vi "Create Measure VI for Client.vi"(7 "client service_class":string, 8 "error in":errorcluster, 9 "results data":T1[](array[typedef]), 10 "configuration data":T4[](array[typedef]), 11 "measure vi refnum":refnum<vi>) -> (0 "error out":errorcluster)   [LabVIEW 2021, in "MeasurementClient Editor.lvlib"]
uses:
  MeasurementClient Editor.lvlib
  <vilib>/gRPC/Generated APIs/ni/measurementlink/measurement/v2/Measurement Service Client/RPC Messages/ni_measurementlink_measurement_v2_ConfigurationParameter.ctl
  <vilib>/gRPC/Generated APIs/ni/measurementlink/measurement/v2/Measurement Service Client/RPC Messages/google_protobuf_Field_Kind.ctl
  <vilib>/gRPC/Generated APIs/ni/measurementlink/measurement/v2/Measurement Service Client/RPC Messages/ni_measurementlink_measurement_v2_ConfigurationParameter_AnnotationsEntry.ctl
  <vilib>/gRPC/Generated APIs/ni/measurementlink/measurement/v2/Measurement Service Client/RPC Messages/ni_measurementlink_measurement_v2_Output.ctl
  <vilib>/gRPC/Generated APIs/ni/measurementlink/measurement/v2/Measurement Service Client/RPC Messages/ni_measurementlink_measurement_v2_Output_AnnotationsEntry.ctl
  <vilib>/gRPC/Generated APIs/ni/measurementlink/measurement/v2/Measurement Service Client/Measurement Service Client.lvlib
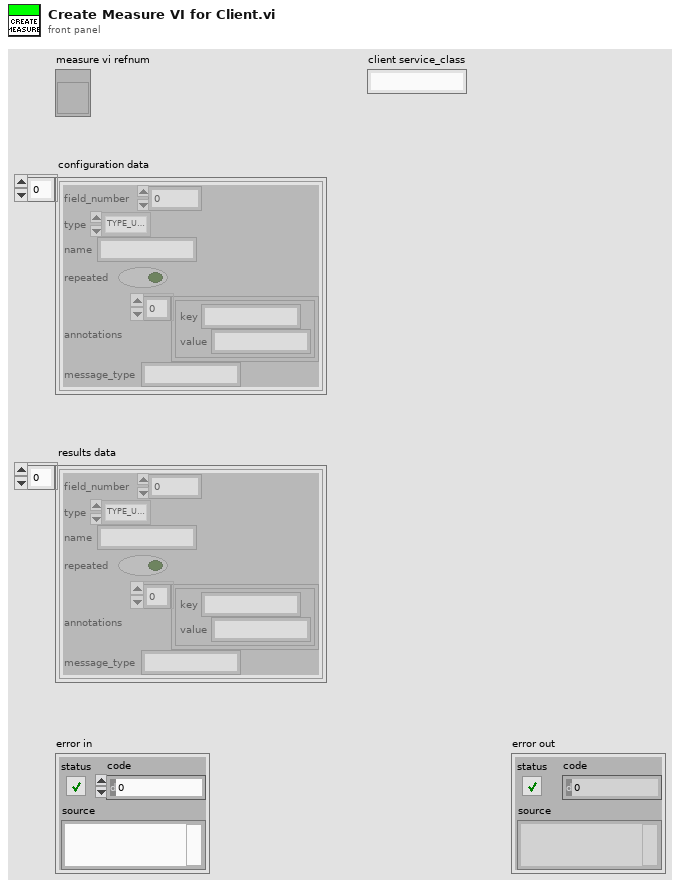
[diagram p1: front panel]
types:
  T1 = typedef "ni.measurementlink.measurement.v2.api.lvlib/Measurement Service Client.lvlib/ni_measurementlink_measurement_v2_Output.ctl" = cluster{"field_number":i32, "type":T2, "name":string, "repeated":bool, "annotations":T3[], "message_type":string}
  T2 = typedef "ni.measurementlink.measurement.v2.api.lvlib/Measurement Service Client.lvlib/google_protobuf_Field_Kind.ctl" = enum32{"TYPE_UNKNOWN", "TYPE_DOUBLE", "TYPE_FLOAT", "TYPE_INT64", "TYPE_UINT64", "TYPE_INT32", "TYPE_FIXED64", "TYPE_FIXED32", "TYPE_BOOL", "TYPE_STRING", "TYPE_GROUP", "TYPE_MESSAGE", "TYPE_BYTES", "TYPE_UINT32", "TYPE_ENUM", "TYPE_SFIXED32", "TYPE_SFIXED64", "TYPE_SINT32", "TYPE_SINT64"}
  T3 = typedef "ni.measurementlink.measurement.v2.api.lvlib/Measurement Service Client.lvlib/ni_measurementlink_measurement_v2_Output_AnnotationsEntry.ctl" = cluster{"key":string, "value":string}
  T4 = typedef "ni.measurementlink.measurement.v2.api.lvlib/Measurement Service Client.lvlib/ni_measurementlink_measurement_v2_ConfigurationParameter.ctl" = cluster{"field_number":i32, "type":T2, "name":string, "repeated":bool, "annotations":T5[], "message_type":string}
  T5 = typedef "ni.measurementlink.measurement.v2.api.lvlib/Measurement Service Client.lvlib/ni_measurementlink_measurement_v2_ConfigurationParameter_AnnotationsEntry.ctl" = cluster{"key":string, "value":string}
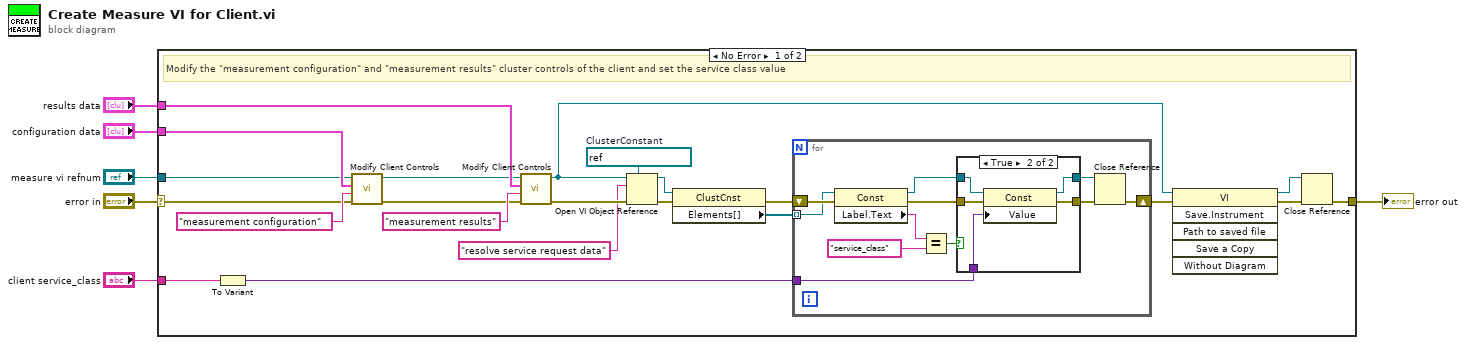
[diagram p0: block diagram]
diagram:
  n1 = case shown="No Error" "error in" {
    selector: "error in" -> [w21 w47]
    tunnel: "configuration data" -> [w28 _]
    tunnel: "results data" -> [w24 _]
    tunnel: "measure vi refnum" -> [w20 _]
    tunnel: [w17 w47] -> w4
    tunnel: "client service_class" -> [w8 _]
    frame No Error {
      w15 = refnum<vi> refnum  # ClusterConstant
      # "Modify the \"measurement configuration\" and \"measurement results\" cluster controls of the client and set the service class value"
      n2 = To Variant(anything=w8) -> (Variant=w7:variant)
      n3 = call "Modify Client Controls.vi"("error in"=w21, "control name"="measurement configuration", "parameter data"=w28, "vi refnum"=w20) -> ("error out"=w26:errorcluster, "vi refnum out"=w23:refnum<vi>)  [unwired: 6 in]
      n4 = call "Modify Client Controls.vi"("error in"=w26, "control name"="measurement results", "parameter data"=w24, "vi refnum"=w23) -> ("error out"=w22:errorcluster, "vi refnum out"=w13:refnum<vi>)  [unwired: 6 in]
      n5 = Open VI Object Reference(7:w15, 8:w22, 10:"resolve service request data" ("name/order"), 11:w13) -> (0:w16:errorcluster, 3:w14:refnum<vi>)
      n6 = property class="ClustCnst"(reference=w14, error in=w16) -> (error out=w11:errorcluster, "Elements[]"=w9:refnum<vi>[])  [unwired: 1 out]
      n7 = for {
        shift-right: [w32] -> w10
        shift-left: w11 -> [w39]
        tunnel: w9 -> [w38] mode=indexing
        tunnel: w7 -> [w30]
        n8 = property class="Const"(reference=w38, error in=w39) -> (reference out=w33:refnum<vi>, error out=w34:errorcluster, "Label.Text"=w37:string)
        n9 = Equal?(x=w37, y="service_class") -> (x = y?=w35:bool)
        n10 = case shown="True" w35 {
          tunnel: w34 -> [w40 w46]
          tunnel: w33 -> [w41 w44]
          tunnel: [w41 w43] -> w29
          tunnel: [w40 w45] -> w31
          tunnel: w30 -> [_ w42]
          frame False {
          }
          frame True {
            n11 = property class="Const"(reference=w44, error in=w46, "Value"=w42) -> (reference out=w43:refnum<vi>, error out=w45:errorcluster)
          }
        }
        n12 = Close Reference(reference=w29, error in (no error)=w31) -> (error out=w32:errorcluster)
      }
      n13 = invoke class="VI" method="Save.Instrument"(reference=w13, error in=w10) -> (reference out=w19:refnum<vi>, error out=w18:errorcluster)  [unwired: 4 in, 4 out]
      n14 = Close Reference(reference=w19, error in (no error)=w18) -> (error out=w17:errorcluster)
    }
    frame Error {
      # "Pass"
    }
  }
  "error out" <- w4
